vi "UHR-Fleezers Control (host) - 11.9b.vi"() -> ()   [LabVIEW 2014] (continued)
  out "Ave. Time (s)":dbl=7.5
  out "1 Channel":waveform(dbl)(graph)={"t0"=timestamp(0 s since 1904-01-01), "dt"=1.4999999999999999e-05, "Y"=array[20000 elements], "attributes"=variant("NI_ChannelName"=variant(string "T1 X"))}
  out "Slow mean":dbl=-0.0035457890155310146 format="%0.2f"
  in  "Slow mean N ave.":dbl=1.0 min=1.0 step=1.0
  out "Mean Intensity":dbl=-0.0035457890155310237
  out "Sigma":dbl=0.00558974165957254
  out "Sigma/Mean":dbl=-1.5764450831926926
  in  "Subtract mean":bool
  in  "High Res. Display":u16(ring)=1 items=["T1 Y", "T1 X", "T1 Sum", "T2 Y", "T2 X", "T2 Sum", "T1 FB X", "T1 FB Sum", "T2 FB X", "T2 FB Sum", "PSD Y", "PSD X", "PSD Y Sum"]
  out "APD 1 Rate (Hz)":dbl format="%#_3p"
  in  "Tab Control":T4(tab)
  in  "Red Laser ON/Interlacing":bool
  out "Good tether":bool
  out "Bad fit":bool
  in  "11":bool
  out "Stage Moving":bool
  in  "Read Cal":bool
  in  "Confocal\nLinescan":bool
  in  "Speed (nm/s)":dbl=100.0
  in  "Furthest Withdraw (MHz)":dbl=15.0
  in  "Confocal\nImage":bool
  in  "Round T1 X":bool caption="Round"
  in  "T1 offset_x (mV)":dbl=-22.37819181637641 format="%#_2g"
  in  "T1 k_x (pN/nm)":dbl=0.15700163781152213 min=0.0 step=0.001 format="%#_2g"
  out "Total Time (s)":dbl=60.0
  in  "Start Saving":bool
  in  "Cal sets to save":u32=25 min=1 step=1
  in  "Comment (data description)":string="testing confocal setup"
  out "Calibrating...":bool
  in  "Trap 2 (ON/OFF)":bool
  in  "Trap 1 (ON/OFF)":bool
  in  "Save Calibration":bool
  in  "N sets to save":u32=200 caption="N Sets"
  in  "Save N Sets":bool
  out "Save file name":path=path "E:/Data/120504/120504_125.dat"
  in  "Save ave N":dbl=250.0 caption="Averaging Factor"
  out "Saving...":bool
  in  "Stop Saving":bool
  out "Progress":u16(slide) scale=0.0..100.0
  out "Manipulating Trap":bool
  out "Buffer Status":dbl(slide) scale=0.0..1.0
  out "Overflow (data lost)":bool
  in  "Reset":bool
  out "Data Rate (Hz)":dbl=66666.66666666667 caption="Trap Data Rate (Hz)" format="%#_3p"
  out "Data Period (s)":dbl=1.4999999999999999e-05 caption="Trap Data Period (s)" format="%#_6p"
  out "Save Data Rate (Hz)":dbl=266.6666666666667 caption="Rate (Hz)" format="%#_6p"
  out "Save Data Period (s)":dbl=0.00375 caption="Period (s)" format="%#_6p"
  in  "T1 a_x (nm/V)":dbl=925.7792512885474 step=10.0 format="%#_3g"
  in  "T2 a_x (nm/V)":dbl=678.0121440160386 step=10.0 format="%#_3g"
  in  "T2 k_x (pN/nm)":dbl=0.2167951647771519 min=0.0 step=0.001 format="%#_2g"
  in  "T2 offset_x (mV)":dbl=-14.421148336697543 format="%#_2g"
  in  "BD 1 Frequency 1 (MHz)":dbl=67.75 caption="T1 X (MHz)" min=60.0 max=90.0 step=1.0 format="%#_6p"
  in  "BD 1 Frequency 2 (MHz)":dbl=83.0 caption="T2 X (MHz)" min=60.0 max=90.0 step=1.0 format="%#_6p"
  in  "Green ON/Interlacing":bool
  in  "Round T2 X":bool caption="Round"
  in  "AO1":dbl(slide)=5.0 caption="Confocal Y (V)" min=0.0 max=10.0 step=0.01 scale=0.0..10.0 scale format="%_1f"
  in  "AO2":dbl(slide)=5.0 caption="Confocal X (V)" min=0.0 max=10.0 step=0.01 scale=0.0..10.0 scale format="%_1f"
  in  "Trap Raster Scan":bool
  out "Raster Scanning...":bool
  in  "Trap D (MHz)":dbl=15.25
  in  "Setpoints (V)":cluster{"Set 1":dbl, "Set 2":dbl}={"Set 1"=9.0, "Set 2"=9.0}
  in  "Green FB Setpoint (mV)":dbl=90.0
  in  "Fish":bool
  out "Multiple tether":bool
  out "Hysteresis":bool
  in  "Target":bool
  in  "Active cal?":bool
  in  "Set Current\nPos to 0,0,0":bool
  in  "Position Label 5":string="Upper flow spot" caption="5"
  in  "Move to Position":bool
  in  "Position":dbl=1.0 min=1.0 max=10.0 step=1.0
  in  "Set Position":bool
  in  "Saved Stage Positions":dbl[][](array[numeric])=[[1.0, 0.0, 0.0, 0.0], [2.0, 0.47143, -1.65361, -0.02271], [3.0, 1.5, -0.5, 0.0], [4.0, -0.17227, -2.30048, -0.0394], [5.0, 1.5, -2.0, -0.02], [6.0, 0.0, 0.0, 0.0], [7.0, 0.0, 0.0, 0.0], [8.0, 0.0, 0.0, 0.0], [9.0, 0.0, 0.0, 0.0], [10.0, 0.0, 0.0, 0.0]]
  in  "Move to Position 5":bool
  in  "z nudge increment (um)":dbl=0.5
  in  "+z":bool
  in  "Position 1 Label":string="Lower capillary (DNA beads)" caption="1"
  in  "Set Position 1":bool
  in  "Set Position 2":bool
  in  "Set Position 3":bool
  in  "Set Position 4":bool
  in  "Move to Position 3":bool
  in  "Move to Position 4":bool
  in  "Move to Position 2":bool
  in  "Move to Position 1":bool
  in  "Position 2 Label":string="Upper capillary (ADig beads)" caption="2"
  in  "Position 3 Label":string="Lower flow spot" caption="3"
  in  "Position 4 Label":string="Dump beads" caption="4"
  in  "-z":bool
  in  "Set Position 5":bool
  out "Stage Control Serial Error":errorcluster
  in  "Use Harvard pumps\nfor beads (else Chemyx)":bool=TRUE
  in  "Tab Control 9":enum32{"Harvard Pumps", "Chemyx Pumps"}(tab)
  in  "Normal volume (mL)":dbl=200.0
  out "Samp flush bar":dbl(slide)=0.8066666666666666 scale=0.0..1.0
  out "Flushing samp":bool caption="Flushing"
  out "P1 Flush Volume (uL)":dbl=100.5 caption="Volume (mL)"
  out "P3 Flush Volume (uL)":dbl=121.0 caption="Volume (mL)"
  out "P3 Flushing Bar":dbl(slide)=0.8066666666666666 scale=0.0..1.0
  in  "Display On P3":bool caption="Display On"
  in  "Normal Flow Rate (ul/h) P3":dbl=800.0 caption="Normal Flow Rate (ml/h)"
  out "Flushing P3":bool caption="Flushing"
  in  "Retract Vol 1 (uL)":dbl=50.0 caption="Volume (mL)"
  in  "Retract Vol 3 (uL)":dbl=100.0 caption="Volume (mL)"
  in  "Retract Rate (mL/m)":dbl=2000.0
  in  "Retract Pump 1":bool
  in  "Retract Pump 3":bool
  in  "Stop Flow":bool
  in  "Start Flow":bool
  in  "Flush Sample":bool
  in  "Flush volume (mL)":dbl=100.0
  in  "Flush rate (mL/m)":dbl=100.0
  in  "Normal Flow rate (mL/h)":dbl=100.0
  in  "Clear Volume":bool caption="Clear Infused Volume"
  in  "Flush Pump 3":bool
  in  "Volume (uL) P3":dbl=150.0 caption="Volume (mL)"
  in  "Flush rate (uL/m) P3":dbl=100.0 caption="Rate (mL/m)"
  out "Flushing P1":bool caption="Flushing"
  in  "Volume (uL) P1":dbl=100.0 caption="Volume (mL)"
  in  "Flush rate (uL/m) P1":dbl=100.0 caption="Rate (mL/m)"
  in  "Normal Flow Rate (ul/h) P1":dbl=600.0 caption="Normal Flow Rate (ml/h)"
  in  "Flush Pump 1":bool
  in  "Clear Volume P3":bool caption="Clear Infused Volume"
  in  "Clear Volume P1":bool caption="Clear Infused Volume"
  in  "Display On P1":bool caption="Display On"
  out "P1 Flushing Bar":dbl(slide)=1.005 scale=0.0..1.0
  out "Samp Volume (uL)":dbl caption="Volume (mL)"
  out "Total Volume\nFlowed P1 (uL)":dbl caption="Total Volume\nFlowed (mL)"
  out "Total Volume\nFlowed P3 (uL)":dbl caption="Total Volume\nFlowed (mL)"
  out "Total Volume\nFlowed Samp (uL)":dbl caption="Total Volume\nFlowed (mL)"
  in  "All Pump Parameters":T5={"Pump 1"={"Diameter (mm)"=4.61, "Units"=4.0, "Volume"=100.0, "Rate"=25.0}, "Pump 2"={"Diameter (mm)"=4.61, "Units"=3.0, "Volume"=0.0, "Rate"=0.0}, "Pump 3"={"Diameter (mm)"=4.61, "Units"=4.0, "Volume"=100.0, "Rate"=800.0}}
  in  "Total Volume\nFlushed (uL)":dbl
  in  "Inject Pump 2":bool caption="Inject Pump 2\n(Flush Center)"
  in  "Flush Center Ch Rate (ul/m)":dbl=100.0
  in  "Flush Center Ch Volume (uL)":dbl=15.0
  in  "Pump pause delay (ms)":u32
  in  "Pump write delay (ms)":dbl=300.0
  in  "Ch 3 Inject Rate (ul/h)":dbl=800.0
  in  "Ch 3 Inject Volume (uL)":dbl=100.0
  in  "Ch 1 Inject Volume (uL)":dbl=100.0
  in  "Ch 1 Inject Rate (ul/h)":dbl=25.0
  out "Pump 1 cont disp":string="Right: DNA beads "
  out "Pump 3 cont disp":string="Left: ADig beads"
  in  "Read Harvard":bool
  out "read buffer":string
  out "Serial Settings:Number of Bytes at Serial Port":u32
  in  "write buffer":string
  in  "Tab Control 2":T6(tab)=enum."Feedback on Trap Position"
  out "Total Counts (ticks)":u32=600
  in  "Trap ON/OFF X or Y Amp?":bool=TRUE
  in  "Oscillate Set 1":bool
  in  "Trap 1 ON":bool
  in  "Number Interlace Sets":u8=3 min=1 max=3
  in  "DIO count 3 (ticks)":u32=200
  in  "DIO count 2 (ticks)":u32=200
  in  "DIO count 1 (ticks)":u32=200
  in  "BD 2 Amplitude 3 (%)":dbl min=0.0 max=50.0 step=1.0
  in  "BD 2 Amplitude 2 (%)":dbl min=0.0 max=50.0 step=1.0
  in  "BD 2 Amplitude 1 (%)":dbl min=0.0 max=50.0 step=1.0
  in  "BD 1 Amplitude 3 (%)":dbl min=0.0 max=50.0 step=1.0
  in  "BD 1 Amplitude 2 (%)":dbl=35.0 min=0.0 max=50.0 step=1.0
  in  "BD 1 Amplitude 1 (%)":dbl=10.0 min=0.0 max=50.0 step=1.0
  in  "BD 2 Frequency 3 (MHz)":dbl=26.0 min=0.0 max=40.0 step=1.0 format="%#_6p"
  in  "BD 1 Frequency 3 (MHz)":dbl=70.0 min=60.0 max=90.0 step=1.0 format="%#_6p"
  in  "BD 2 Frequency 2 (MHz)":dbl=26.0 min=0.0 max=40.0 step=1.0 format="%#_6p"
  in  "BD 2 Frequency 1 (MHz)":dbl=26.0 min=0.0 max=40.0 step=1.0 format="%#_6p"
  in  "Not-Interlacing Set":enum32{"Set 1", "Set 2", "Set 3"}(radio)
  in  "Interlace":bool=TRUE
  in  "Trap 2 ON":bool
  in  "Trap 3 ON":bool
  in  "Scan axis 2":bool=TRUE
  in  "Osc. freq. (Hz)":dbl=0.25
  in  "Osc. amp. (MHz)":dbl=2.0
  out "Coords":T7
  in  "Manipulation Scaling":cluster{"Horizontal":dbl, "Vertical":dbl}={"Horizontal"=0.075, "Vertical"=0.01}
  in  "Freq or Amp switch first":bool=TRUE
  in  "Swap F1 and F2":bool
  in  "Freq switch delay":u16
  in  "Amp switch delay":u16=5
  in  "MCL Step Increment (V_int)":dbl=3.0
  out "Time to Finish All (min)":dbl=0.15651 format="%#_2p"
  in  "Scan Speed (nm/s)":dbl=100.0
  in  "Scan Range (nm)":dbl=470.0
  in  "Step Size (nm)":dbl=1.0
  in  "MCL/AOM Scale Tweak":dbl=1.0
  in  "MCL Step Position Ratio":dbl=0.5
  in  "Move MCL Also?":bool=TRUE
  out "Final sep (nm)":dbl=1520.75
  out "Initial sep (nm)":dbl=1050.75
  out "Save index":dbl=125.0
  out "Final D (MHz)":dbl=19.071138211382113
  out "Initial D (MHz)":dbl=15.25
  out "Final freq. (MHz)":dbl=63.92886178861789
  out "Initial freq. (MHz)":dbl=67.75
  in  "Saved AOD Raster Scan Parameter Sets":T8(array[cluster])=[{"Scan Range AOD (nm) 2"=500.0, "Step Size AOD (nm) 2"=1.0, "Scan Speed AOD (nm/s) 2"=100.0, "Number of scans (AOD) 2"=1, "Label"="offset curve"}, {"Scan Range AOD (nm) 2"=450.0, "Step Size AOD (nm) 2"=1.0, "Scan Speed AOD (nm/s) 2"=100.0, "Number of scans (AOD) 2"=1, "Label"="hp raster check"}, {"Scan Range AOD (nm) 2"=6.8, "Step Size AOD (nm) 2"=0.34, "Scan Speed AOD (nm/s) 2"=0.34, "Number of scans (AOD) 2"=1, "Label"="3.4 kbp - 1 bp steps"}, {"Scan Range AOD (nm) 2"=215.0, "Step Size AOD (nm) 2"=1.0, "Scan Speed AOD (nm/s) 2"=100.0, "Number of scans (AOD) 2"=3, "Label"="dt14 1 14 MHz start"}, {"Scan Range AOD (nm) 2"=450.0, "Step Size AOD (nm) 2"=1.0, "Scan Speed AOD (nm/s) 2"=100.0, "Number of scans (AOD) 2"=1, "Label"="dt14 2 small beads"}, {"Scan Range AOD (nm) 2"=470.0, "Step Size AOD (nm) 2"=1.0, "Scan Speed AOD (nm/s) 2"=100.0, "Number of scans (AOD) 2"=1, "Label"="Oligo"}, {"Scan Range AOD (nm) 2"=410.0, "Step Size AOD (nm) 2"=1.0, "Scan Speed AOD (nm/s) 2"=100.0, "Number of scans (AOD) 2"=1, "Label"="hp raster check"}, {"Scan Range AOD (nm) 2"=650.0, "Step Size AOD (nm) 2"=1.0, "Scan Speed AOD (nm/s) 2"=100.0, "Number of scans (AOD) 2"=1, "Label"="Monika"}, {"Scan Range AOD (nm) 2"=1000.0, "Step Size AOD (nm) 2"=1.0, "Scan Speed AOD (nm/s) 2"=100.0, "Number of scans (AOD) 2"=1, "Label"="Monika offset"}]
  in  "Load parameters":bool
  out "Scan Range (MHz)":dbl=-3.821138211382114
  in  "Restart DMA? (AOD)":bool=TRUE caption="Restart DMA?"
  out "Incr. int (AOD)":i64=-7759651845
  out "Time/Scan (s) (AOD)":dbl=4.6953000000000005 format="%#_2p"
  out "Data points/scans":dbl=626040.0
  out "Data points/scan (f/b)":dbl=626040.0
  in  "Save scans":bool=TRUE
  out "AOD Scan I":u64 caption="Scan I"
  in  "Continuous AOD Scanning":bool caption="Continuous Scanning"
  in  "Abort AOD Scan":bool caption="Abort Scan"
  in  "Scan BD":bool=TRUE
  out "Cycles/step (AOD)":u64=666 format="%.3p"
  in  "Number of F/B Scans (AOD)":u16=1 min=1
  out "Scan steps (AOD)":u64=470
  out "Scan Increment (MHz)":dbl=-0.00814741622895973
  out "AOD Scanning":bool caption="Scanning"
  in  "Start AOD Scan":bool caption="Start Scan"
  out "N sets should be saved":dbl=31.302
  out "Progress 2":u16(slide) caption="Progress" scale=0.0..100.0
  in  "Abort save 2":bool caption="Abort save"
  in  "Trap 1 Bead Size (nm)":dbl=860.0
  in  "Trap 2 Bead Size (nm)":dbl=790.0
  out "MCL Count":dbl=782931.6080202644
  in  "All FB On/Off":bool=TRUE
  in  "AI2 to Setpoint":cluster{"Set 1":bool, "Set 2":bool}
  out "AI2 (V)":cluster{"Set 1":dbl, "Set 2":dbl}={"Set 1"=-0.0027466658528397473, "Set 2"=-0.0030518509475997192}
  in  "Reset Feedback":cluster{"Set 1":bool, "Set 2":bool}
  in  "PID Gains":T9={"Set 1"={"proportional gain (Kc)"=0, "integral gain (Kc*Ts/Ti)"=5, "derivative gain (Kc*Td/Ts)"=0}, "Set 2"={"proportional gain (Kc)"=0, "integral gain (Kc*Ts/Ti)"=5, "derivative gain (Kc*Td/Ts)"=0}}
  in  "Feedback On/Off":cluster{"Set 1":bool, "Set 2":bool}={"Set 1"=TRUE, "Set 2"=TRUE}
  in  "Rem fb disp offset":bool caption="Rem. Offset"
  in  "Remove Offset to factor":bool
  in  "FB Trap Pos Offset":dbl=-9.744913000168507 caption="Offset (nm)" format="%.1f"
  in  "Negate Y Axis":bool=TRUE
  in  "Set Reading to\nSetpoint":bool
  out "Trap X (AI1)":T10={"Trap 1"=0.29998779296875, "Trap 2"=0.399993896484375}
  in  "Trap Pos FB SP":fxp<+/-,16,1>=-0.10723876953125 caption="Setpoint"
  in  "Trap Pos. FB ON":bool
  in  "Reset Trap Pos. FB":bool
  out "Trap Positions":waveform(dbl)[](graph)=[{"t0"=timestamp(13.800000000000011 s since 1904-01-01), "dt"=0.15, "Y"=[-9.744913000165011, -9.744913000165011], "attributes"=variant("NI_ChannelName"=variant(string "Trap 1 Pos."))}, {"t0"=timestamp(13.800000000000011 s since 1904-01-01), "dt"=0.15, "Y"=[-3.495870259939693e-12, -3.495870259939693e-12], "attributes"=variant("NI_ChannelName"=variant(string "Trap 2 Pos."))}]
  in  "Tab Control 8":enum32{"Main Setting", "Details"}(tab)=enum."Details"
  in  "Green Laser ON/OFF":bool
  in  "Offset SP2 from SP1":bool
  in  "Use SP 2":bool
  in  "Trap Pos FB Int Count":u16=100
  in  "Trap Pos. FB Gains":T11={"proportional gain (Kc)"=10.0, "integral gain (Kc*Ts/Ti)"=10.0, "derivative gain (Kc*Td/Ts)"=0.0} {"proportional gain (Kc)" format="%.11g"; "integral gain (Kc*Ts/Ti)" format="%.11g"; "derivative gain (Kc*Td/Ts)" format="%.11g"}
  in  "Trap Pos FB SP 2":fxp<+/-,16,1>=-0.10723876953125 caption="Setpoint 2"
  in  "SP2 Offset":fxp<+/-,16,1>=0.100006103515625
  in  "Negate Diff?":bool=TRUE
  in  "Differential FB?":bool=TRUE
  in  "Trap Pos. FB Offset Factor":i64
  in  "Trap Pos FB Negate Action":bool
  in  "Trap Pos. FB Mult Factor":i64=16777216
  in  "Trap Pos. AI1 X Pre-scale":u16
  in  "Trap Pos. FB Range":T12={"output high"=0.999969482421875, "output low"=-1.0}
  out "Trap Pos FB Int Signal":fxp<+/-,24,9>=-2.007537841796875 format="%.18g"
  out "Trap Pos FB Int-Norm Signal":fxp<+/-,16,1>=-0.02008056640625 format="%.16g"
  in  "Set SP Using...":bool
  in  "Trap Pos FB Monitor\nT1 or T2":bool
  out "Trap X AI1 (DMA)":T13={"Set 1"=-1.0, "Set 2"=-1.0}
  in  "N El. to Ave.":dbl=10000.0
  out "Trap Pos FB Action":i64
  out "Action (%)":dbl(knob) scale=-100.0..100.0
  in  "Trap Pos. FB Out Scale 2^n":u8=24 caption="Action Scale Factor"
  out "Mean T1 Position (nm)":dbl=-9.744913000165011 caption="Mean T1 (nm)" format="%0.2f"
  out "Trap 1 Position RMS (A)":dbl caption="RMS (Å)"
  in  "Remove Action Offset":bool
  in  "factor":dbl=0.8
  in  "Trap Pos. Disp. Downsample":dbl=10000.0 caption="Trap Downsample"
  in  "Tab Control 3":enum32{"Timing", "MCL Scan", "Analog Out"}(tab)
  out "APD 2 Gate Late Counter":u32
  out "APD 2 Gate Relative Phase":i16
  in  "Phase Adj. (APD 2 Gate)":i16=20
  in  "Initial Phase Adjustment (APD 2 Gate)":i16=55
  out "APD 1 Gate Late Counter":u32
  in  "- phase (APD 1 Gate)":bool
  in  "+ phase (APD 1 Gate)":bool
  out "APD 1 Gate Relative Phase":i16
  in  "Phase Adj. (APD 1 Gate)":i16=20
  in  "Initial Phase Adjustment (APD 1 Gate)":i16=60
  in  "Save APD Data\nwith Trap Data":bool=TRUE
  out "APD FIFO Elements Remaining":u32
  in  "- phase (APD Acq)":bool
  in  "+ phase (APD Acq)":bool
  out "APD Acq Late Counter":u32
  out "APD Acq Relative Phase":i16
  in  "Phase Adj. (APD Acq)":i16=20
  in  "Initial Phase Adjustment (APD Acq)":i16
  in  "Invert APD Gate":bool caption="Invert Gate"
  in  "APD Gate OFF Count":u32=450 caption="Gate OFF Count"
  in  "APD Gate ON Count":u32=150 caption="Gate ON Count"
  in  "APD Gate":enum32{"ON", "OFF", "Interlace"}(radio)=enum."Interlace"
  in  "APD Integration Time (s)":dbl=0.01 caption="Integration Time (s)"
  out "APD Acq Rate (Hz)":dbl=100.0 caption="Rate (Hz)"
  out "APD Samples/FIFO Acq.":dbl=30.0
  out "APD Elements/DMA read":u32=60
  out "APD Int. Count":u32=400000 format="%.0p"
  in  "+ phase (APD 2 Gate)":bool
  in  "- phase (APD 2 Gate)":bool
  in  "Tab Control 5":enum32{"PSD X", "PSD Y", "Other Data Channel"}(tab)
  out "Data map":dbl[][](graph)=[[-0.009093117685790525, -0.007930362371143508, -0.007754257275205968, -0.008007549817249278, -0.007602052846338941, -0.007912268435502932, -0.007607960084622785, -0.0075511280459739025, -0.0075659235273027765, -0.008250603527173198, -0.00813251622962637, -0.008594668588708203, -0.009399585249933565, -0.007647222257289099, -0.009101202856383231, -0.008282046280890548, -0.009811094602988905, -0.00756717949318091, -0.009140567007915868, -0.0073843309806302946], [-0.008493807361303536, -0.007663617072649492, -0.008256205022532336, -0.007952830185196302, -0.007279874418184582, -0.007356798116565186, -0.0069743489143222585, -0.007520087991651134, -0.007361850724229795, -0.007389116586560407, -0.007775790827289851, -0.008683184943784783, -0.008790211727097149, -0.007806810616736395, -0.008982907777700291, -0.007650155522875499, -0.009388247877714903, -0.007552137445539828, -0.008977826950618533, -0.007886203299123228], [-0.008181893320929307, -0.00839471338042945, -0.007799952401828855, -0.008308044384906312, -0.008275645030715005, -0.007401990323496574, -0.006875323319245371, -0.0070218178801166025, -0.006512198698798073, -0.0063178688570392095, -0.006805180239267433, -0.007518346532565596, -0.008735692049743055, -0.00724608634970231, -0.008704712767052859, -0.007945321438686287, -0.008767860926849669, -0.007671020451478872, -0.00875386344445876, -0.007695295089867138], [-0.008130119935988365, -0.007136557696350718, -0.007373598169435823, -0.007233072138047845, -0.0077281747998472865, -0.005849249829228351, -0.005735947777185798, -0.004739559736975043, -0.004920183410197928, -0.0038166885698606785, -0.004682785911972345, -0.005039020484130334, -0.00690087468071523, -0.006215680179303547, -0.0074666456406588646, -0.00814641889723231, -0.008228414513586805, -0.0073042911866212775, -0.008535443147109325, -0.007689317045800068], [-0.008048339688765222, -0.0070262103984282814, -0.006784428381835994, -0.006462947020101757, -0.005413544226518168, -0.0028972309457726553, -0.002613656344091552, -0.0007913579983610413, -0.0010255539568848066, 0.0006448033640966027, -0.0005086805713629527, -0.001297083649014534, -0.003337801791559313, -0.002740630934904912, -0.005540289041049259, -0.006466196037469115, -0.007893084684782161, -0.007253383480927094, -0.008523649067154491, -0.008424970867227096], [-0.008692622082261615, -0.007319521217364842, -0.005755111221817798, -0.003792540532687189, -0.00227942708102312, 0.000483266681506554, 0.0014973802606671, 0.003540650121447641, 0.004028332480785218, 0.005135244197648001, 0.003981153966581634, 0.0034636396067710545, 0.0017501855516850323, 0.0010275870097429896, -0.0024058090542775825, -0.004619508847101628, -0.00696689371632374, -0.006931245628688383, -0.008182025780859851, -0.007815950695329976], [-0.00821540874240863, -0.005867179558433026, -0.0038147206017466926, -0.0012540547752299272, 0.0009272510857660976, 0.004482725069077296, 0.005094761342461562, 0.006396333111961989, 0.006641489865394995, 0.008244873838360105, 0.00622024214014944, 0.005437421631898459, 0.0037062196383043787, 0.0039079284440514134, 0.00011910739683561111, -0.0021155745359372523, -0.0052920825878262235, -0.006269707480838847, -0.00771057032521053, -0.007948241106374241], [-0.007884864746179087, -0.005659354512526344, -0.002544916655066751, 9.730381565131179e-05, 0.0019679392499950933, 0.003980498813834972, 0.004545595176909105, 0.005211998880279077, 0.004316308793345271, 0.0049582106101100296, 0.004417272839063756, 0.004152457319364951, 0.0028044785889019025, 0.00406546833676348, 0.0004537962268733079, -0.0022503305680760134, -0.004833591485740649, -0.005815590438963289, -0.006409661910137404, -0.00747004429812991], [-0.007583267382238386, -0.004882000882934762, -0.0038451140355032776, -0.0016369446668547012, -0.0012364145574272002, 0.00024560570156679373, 0.0001795553469662146, 0.00059301095989026, -0.0004598253721832719, 0.0006432265077103554, -0.0005366492251270509, -0.00024492525087133033, -0.0008478979763931471, 0.0004355022865183716, -0.002224596882477229, -0.0030354619889501723, -0.005565311948490649, -0.006021505826488022, -0.0069210753467628845, -0.007879944918476524], [-0.008040346878090326, -0.006862696971498104, -0.006336491878674995, -0.005461350586097968, -0.005940054654849293, -0.004512649878881008, -0.005018950037994686, -0.0043380418634407164, -0.004709873373528969, -0.004442153494476381, -0.005131912732517138, -0.004937093503234647, -0.006064322362111088, -0.004728773424951794, -0.006301422293530947, -0.006624384767080079, -0.008081381277763696, -0.00789390592402444, -0.007979806702532219, -0.007895618667850521], [-0.009072596458312808, -0.00880289426096623, -0.0092848563929495, -0.010326479907538676, -0.010798822549107683, -0.009119956258571284, -0.009276114327973069, -0.009089354383039431, -0.009417098163877372, -0.009282915028834361, -0.010344781966702844, -0.009775595105550903, -0.010376003571655317, -0.01021568866775812, -0.011229840225717491, -0.010464341733335863, -0.010657278856759583, -0.009430048577759108, -0.009007295643070796, -0.008342923163363568], [-0.010032577110923473, -0.01048419830062017, -0.01247741022526665, -0.013958311167976727, -0.014919942316729927, -0.014408175422791913, -0.014103923396234723, -0.014744110243936143, -0.014993684986384455, -0.014308447607056084, -0.014937884607659595, -0.015720355253606696, -0.01581234985152132, -0.015517778210244481, -0.01570381347938231, -0.014005181025264823, -0.012564060007705888, -0.01019230034187177, -0.00996108339473993, -0.009007894716188836], [-0.01015831765102569, -0.011625066910300597, -0.013873555893446923, -0.01642046988438768, -0.01850466093024781, -0.019125349960614338, -0.018875498399497426, -0.018924030983383168, -0.02003782808665338, -0.019680135464925662, -0.0199962216477468, -0.02075322752078982, -0.021393804340805025, -0.01892377236854445, -0.017709124629425012, -0.015373965133689256, -0.012883748138151182, -0.011135266972937988, -0.01001563256802752, -0.009346177295655143], [-0.010235131581835623, -0.010548350660948624, -0.01319737955485069, -0.0170756093956873, -0.019682853747901498, -0.021422463301004592, -0.023065732990637723, -0.02311157923810582, -0.02400703774239577, -0.024058458246623678, -0.0240676102995906, -0.02454338695921686, -0.023059059168390954, -0.02006456011149576, -0.017542880027533084, -0.015594551823595627, -0.012758502028002598, -0.010692028843963627, -0.009120734769953582, -0.009382803853976038], [-0.00927124611976432, -0.010163129942715295, -0.012001835840693881, -0.015492617365098072, -0.01804371733697946, -0.020276281639691262, -0.02249444284045994, -0.02399581278990765, -0.02410995799246074, -0.024520143091590986, -0.024440837449861495, -0.023755329314732447, -0.02173444185100297, -0.01888988196650751, -0.015717316137677406, -0.01330102590922941, -0.010307393064907727, -0.009992927689312977, -0.008948368344090785, -0.009171185426330289], [-0.008913670110033758, -0.009487748541153324, -0.010271220953760277, -0.012822685168547666, -0.014877933408246618, -0.01645708382270735, -0.018174418710522888, -0.02006592401438696, -0.020560245735494094, -0.020880445185878234, -0.019757749059474437, -0.019731420523350106, -0.01748349679551805, -0.014933401179938435, -0.01287075469100105, -0.012375615253101852, -0.01017571614409014, -0.010194053140322132, -0.008327555288192647, -0.009296945225881956], [-0.008651703429240758, -0.00859123261526902, -0.0087124516001243, -0.010702988201589679, -0.011158446775450175, -0.013551662787714375, -0.013899713264433188, -0.015139676175909094, -0.015358154174100445, -0.01585371404194936, -0.015240285383275445, -0.015633640866232926, -0.013444202320888608, -0.012235117407072522, -0.010180277760900221, -0.010599065418614181, -0.008836891782999633, -0.009612080137946436, -0.008061008352690049, -0.008692954060992533], [-0.008978999428748309, -0.00853630494854542, -0.008448003588981772, -0.009555269362758849, -0.009800170309108366, -0.010532180047368476, -0.011577191415346372, -0.012522786451981825, -0.011897509550792433, -0.012765293465086206, -0.012382882546317676, -0.012580658559524002, -0.011517787256641054, -0.011479669503957436, -0.009468386619803586, -0.009506617110587617, -0.008814998176882461, -0.008907308155253858, -0.008359272542371161, -0.007728018696215012], [-0.008567772547654876, -0.009179160254178084, -0.008797883700935975, -0.008966540233807333, -0.009244399721063817, -0.010241100172431, -0.009683978551547411, -0.010741416747860222, -0.010801534838144658, -0.011948471067133912, -0.010638943408897612, -0.011276692781352033, -0.010482972789145662, -0.009951530542563796, -0.008872861351211857, -0.009011466300733673, -0.008130228774171959, -0.008497529899096853, -0.008537094090014226, -0.008554927038672385], [-0.00883740874692164, -0.008522568147033945, -0.008057007463930647, -0.00857500256200953, -0.00892333639038801, -0.0102483493423614, -0.009382806505145502, -0.010288681907090315, -0.009776552705287204, -0.010709303069246771, -0.009812157424141538, -0.011540991338011664, -0.009448072118884751, -0.009215522072108621, -0.007990643964211522, -0.00861551413050941, -0.008069591988205893, -0.008448705150511306, -0.008173872666663988, -0.0077366764957025325], [-0.00866188543514634, -0.00837290321697088, -0.007616576548930206, -0.008620554974306619, -0.008879342477325386, -0.009976131360122594, -0.009197328720787731, -0.010891970058339532, -0.009831409253817102, -0.010963285150790543, -0.00943682713188495, -0.010250758011437967, -0.009316627581118588, -0.008698498423952166, -0.007894210972856612, -0.008627558747470431, -0.008684295707717409, -0.008540742057574494, -0.008058236803640907, -0.008796687176971204], [-0.008960243147743728, -0.008389810955552138, -0.00847348274282588, -0.008961453295347137, -0.008457770304110886, -0.00929036551389055, -0.008754051280419149, -0.010523443067409842, -0.009918731765266534, -0.010037112915448395, -0.0094884291794276, -0.009837286274472896, -0.008576890056086488, -0.008579749000379288, -0.0076704608190795035, -0.008975965021771925, -0.00787633064191945, -0.008529814016465537, -0.008210449633173293, -0.00923149421792313], [-0.008958509491948936, -0.0079752458499608, -0.007575580767324844, -0.008803256661217552, -0.008651176181790142, -0.009290225911366488, -0.008694199017275235, -0.00928758206050638, -0.008685080197252814, -0.009895043342157074, -0.008890181034455161, -0.009708286739414866, -0.008159548355032305, -0.008011065029368486, -0.007472994792829198, -0.008178707159361769, -0.008186872200841244, -0.008748187311294335, -0.008332749653614566, -0.009032986118264676], [-0.008984454676541142, -0.008385860780740762, -0.008233303603375429, -0.008883308711661035, -0.008263391222137696, -0.008615507326621034, -0.008345881820440536, -0.009360059323812333, -0.008525712363877502, -0.00936688813432775, -0.008501006453744242, -0.009857020401666132, -0.008518026774209042, -0.008466286706819728, -0.007595230844466895, -0.008637429843490887, -0.008247148821298463, -0.009757163330206205, -0.008351945487579443, -0.008826303902292224], [-0.008793473634059202, -0.008532826676629766, -0.008301057942882255, -0.007918519844410386, -0.008166427002916622, -0.008334776051627416, -0.008198383116294311, -0.008466661691906446, -0.008900494330306541, -0.009018032342304892, -0.008921561030554092, -0.00970008519907525, -0.00858060303466588, -0.008488668571179206, -0.008067629578802802, -0.009301914211857531, -0.007584888207047696, -0.009401246667708162, -0.00838952961198379, -0.009295622811186042], [-0.008612970994324173, -0.009228313227038376, -0.008109777026918365, -0.007900894002180022, -0.008577211653308246, -0.0078092842189432105, -0.009066038409420633, -0.008632114747530527, -0.00915628345868762, -0.009033529956806095, -0.008473548831738616, -0.009753001297439137, -0.008794013472457105, -0.009389760586935149, -0.008294543199585239, -0.009165299461629816, -0.0080445379542478, -0.01003357859191055, -0.008128570719288741, -0.009697938695473063], [-0.00842310878053087, -0.009238538415546935, -0.00789546954167132, -0.007785705695342489, -0.009075128619983087, -0.008134761036174236, -0.009034531715798766, -0.009110522965510081, -0.009372563691683431, -0.00973005869285193, -0.00918442879120475, -0.010224588766867198, -0.009149068560019315, -0.009118548250909013, -0.008665028583165667, -0.009663782970913627, -0.00822885864974483, -0.009561747582651057, -0.007796335718971677, -0.009448741371668462], [-0.008678814702107202, -0.008811871163062448, -0.008591634991878266, -0.008380498253149257, -0.008708521567010137, -0.009080766138792232, -0.009201278029004847, -0.009050300838444577, -0.00961322000266123, -0.009519398380897704, -0.009289741534829938, -0.010063257530557933, -0.009451879246656355, -0.009483739594157017, -0.008678484677225835, -0.00990455006759744, -0.00828239408358521, -0.009970239333168224, -0.008374145539585563, -0.009350844619784601], [-0.008045661641927443, -0.008394412754688788, -0.008552414855659416, -0.009271231425342906, -0.009328147806528048, -0.009046283727420858, -0.009056500460447304, -0.009214165466210778, -0.008945766230968395, -0.009389003022486266, -0.009144492868201123, -0.010147409487001281, -0.009339702713667958, -0.009380077870026074, -0.00835831230057397, -0.009990575898077645, -0.00854232985662241, -0.010366719217208723, -0.008640298575886954, -0.009403613854008858], [-0.008906889127393642, -0.00883118612173188, -0.008453805334277639, -0.00911933095261894, -0.00944887473163078, -0.010310422619086147, -0.009422604595844552, -0.009605385777620547, -0.008426093890224026, -0.01002127148121337, -0.009163459766844236, -0.009814776920437831, -0.008805402929197629, -0.009061616458602838, -0.008487717951513573, -0.009191908002197161, -0.00895972804734331, -0.009660499045960346, -0.008531815925380855, -0.009156879524597247], [-0.008741790054105969, -0.008549257028348849, -0.008797177164368942, -0.009662615006030037, -0.009307487432021831, -0.010322476933490709, -0.008290986210407227, -0.009590805326173235, -0.008934433308237403, -0.009471594992405057, -0.009687824691862398, -0.008931649605826689, -0.008484875544949318, -0.008583409860835651, -0.008351995170223395, -0.009053355535672075, -0.008484405156741804, -0.009874981465109369, -0.008438016030919395, -0.008858275353968496], [-0.00856709491696853, -0.00871265258961926, -0.007921953758409758, -0.009438005293459928, -0.008790640173333714, -0.0093055027234527, -0.008862492730787506, -0.009554208136696149, -0.008482487683988672, -0.01056028798055526, -0.009019149534255914, -0.010050471464200648, -0.00853462219965744, -0.009035449977530046, -0.008112572868495047, -0.008163535201347372, -0.008202407620730396, -0.008747092382002523, -0.00884982609053558, -0.008679668249538044], [-0.008394092371377686, -0.008489154891055648, -0.007659112578658681, -0.00902617957109932, -0.008357595543619473, -0.00961141464742498, -0.008884930906477895, -0.009113321109040815, -0.008880712493923793, -0.010292101237114604, -0.008975496191390358, -0.009710498384115248, -0.008935238162886418, -0.008502221359307316, -0.007752007669347329, -0.007720289124192612, -0.00788689558570684, -0.009181183359262636, -0.00856116046669701, -0.008611585911764589], [-0.008107502655444382, -0.008803676635770773, -0.008830636807290671, -0.008630461742231518, -0.008271369463273916, -0.009203900561491018, -0.008405901304371377, -0.009465853346718931, -0.008950045768193703, -0.009917010857616374, -0.008801581772901624, -0.010150568437297405, -0.008851987437577317, -0.00849255435289463, -0.007881778453429272, -0.007697298607360614, -0.007699527977878644, -0.008589254525886943, -0.007882418667869784, -0.007557576864658732], [-0.008427126089052106, -0.008873246741217405, -0.007984509944572782, -0.008215086829640958, -0.008087204687383241, -0.008627825617963911, -0.008679915351090582, -0.008599184356607833, -0.008277243783790082, -0.009885402202754485, -0.008578730059413158, -0.009265716716539838, -0.008533719952427615, -0.008773683534694161, -0.00758856120767947, -0.008144086881928147, -0.008079560975909644, -0.008313965537627473, -0.008565002742326862, -0.008110889204162412], [-0.008120547360555588, -0.008248284005375792, -0.007905963350631368, -0.008299804257910725, -0.007514734008193604, -0.008466861391934699, -0.007969212201198558, -0.007888984029732645, -0.008696999162581685, -0.009067749176828406, -0.008736340056677103, -0.008654004998204434, -0.008344040713692526, -0.008594741510905897, -0.0074614182850967405, -0.008103078495185257, -0.008057187148527191, -0.008974257694279996, -0.008197872328626302, -0.0074028505391394404], [-0.008307364139471399, -0.00821873274915887, -0.007970649657121935, -0.00815826403385205, -0.008457049180131213, -0.008316579982009714, -0.00790309541305004, -0.007939607987239819, -0.008478315283633124, -0.008288272322383177, -0.009147562816129263, -0.008684972824515615, -0.008675749750533264, -0.007960612097219584, -0.008024961861627669, -0.008590987458143061, -0.007831114204848427, -0.009273090840284501, -0.007678985566660499, -0.008250217200435749], [-0.008439006720363235, -0.008607324538260196, -0.008928480199152027, -0.00907069045095883, -0.008371906943686698, -0.00843318137977436, -0.007928947055533257, -0.008211444982725611, -0.007814800246802284, -0.008561224417862523, -0.0083263104139755, -0.00864694388438663, -0.008317511287294722, -0.008392142509562009, -0.0080180144415389, -0.00841215643506122, -0.008129752772469346, -0.009147606927106531, -0.008461182057229562, -0.008704070030515779], [-0.008805306104753604, -0.008527006486683296, -0.008608832647163441, -0.008197721113858471, -0.008101085524828317, -0.008548783050390606, -0.008327728211326255, -0.00811669551471623, -0.007841959263305661, -0.008369922080743528, -0.007863509709325214, -0.008398594443287834, -0.008357926530931568, -0.007776338967419011, -0.00761957377022411, -0.00797846909846784, -0.00760217145174542, -0.009062943091421194, -0.008736809526389501, -0.009068120509011127], [-0.008594961447082165, -0.00896668650229153, -0.008417303751339367, -0.008410738059004663, -0.008191514788819833, -0.008993325778492794, -0.008023878772254618, -0.008285263880744707, -0.00783265428172105, -0.0073528870683615775, -0.008791245239786302, -0.00865234690848487, -0.008338402850135743, -0.00784027413088714, -0.007823138263178549, -0.007490285631650851, -0.008212733160155018, -0.008264156227590665, -0.008446206631865719, -0.00904272930587351]]
  in  "Channel":i32=4
  in  "Abort MCL Scan":bool
  out "MCL Scan I":u64
  out "MCL Scanning":bool
  in  "Start MCL Scan":bool
  out "wait to reset values":bool
  in  "Tab Control 4":enum32{"Scan Settings", "MCL FPGA Loop Timing"}(tab)
  out "Total Time (s)":dbl=48.0
  in  "Scan lines (y)":u64=20
  in  "Fast Scan Dir":bool=TRUE
  in  "2D or 1D Scan":bool=TRUE
  out "Initial X":dbl=-1.3598098696859644
  out "Initial Y":dbl=6.297618030335399
  out "Time/f+b scan (s) (MCL)":dbl=2.4 caption="Time/scan (s)"
  in  "Number of scans (MCL)":u64=1 caption="Scans"
  in  "Scan steps (MCL)":u64=40 caption="Scan steps (x)"
  in  "N APD Samp/step":dbl=3.0
  in  "Scan Range (V)\n(of steps)":dbl=3.5
  in  "Restart DMA? (MCL)":bool=TRUE caption="Restart DMA?"
  in  "Continuous MCL Scanning":bool caption="Cont. Scanning"
  in  "Center Scan":bool=TRUE
  in  "Save Data (MCL)":bool=TRUE caption="Save Data"
  out "Actual Incr. int (MCL)":i16=294 caption="Incr. int"
  out "Desired incr (int)":dbl=294.0628205128205
  out "Desired Scan Incr (V)":dbl=0.08974358974358974
  out "N sets should be saved (MCL)":dbl=160.0 caption="N sets should be saved"
  out "Data points/scans (MCL)":dbl=4800.0 caption="Data points/scans"
  out "Data points/scan (f+b)":dbl=240.0 caption="points/scan (f+b)"
  out "Cycles/step (MCL)":u64=2000 caption="Cycles/step" format="%.0p"
  out "Actual MCL Inc (V)":dbl=0.08972441785943175
  in  "Phase adjust (MCL)":i16 caption="Phase adjust"
  out "Relative Phase (MCL)":i16 caption="Relative Phase"
  in  "Initial Phase Adj. (MCL)":i16 caption="Initial Phase Adj."
  in  "Update Count (MCL)":u32=600
  in  "+ phase (MCL)":bool
  in  "- phase (MCL)":bool
  out "MCL Late Counter":u32
  in  "APD 1 AO Mult.":i16=1 min=1
  in  "APD 2 AO Mult.":i16=1 min=1
  in  "Red current when FB OFF (%)":dbl
  in  "Tab Control 7":enum32{"Green FB Signals", "Slow MCL Scan"}(tab)
  out "Green FB Plot":dbl(graph)=-0.008239997558519242
  out "MCL Scan 2":cluster{"Begin (V)":dbl, dbl, dbl[]}(graph)
  out "MCL Scan":cluster{"Begin (V)":dbl, dbl, dbl[]}(graph)
  in  "Green laser mode":enum32{"Laser ON", "Laser OFF", "Interlace"}(radio)=enum."Interlace"
  in  "GI Frequency, ON count":u32=150 min=1 step=1
  in  "Invert GI":bool
  out "GI Late Counter":u32
  in  "Phase adj. (GI)":i16=5
  out "GI relative phase":i16
  in  "+ phase (GI)":bool
  in  "Initial Phase Adjustment (GI)":i16=19
  in  "GI Frequency, OFF count":u32=450 min=1 step=1
  in  "- phase (GI)":bool
  out "Green FB Signals (V)":cluster{"Y":dbl, "X":dbl, "Sum":dbl}={"Y"=-1213.5925925925926, "X"=-1213.5925925925926, "Sum"=-0.008239997558519242}
  out "Relative phase (Green FB)":i16
  in  "+ phase (Green FB)":bool
  in  "- phase (Green FB)":bool
  out "Green FB Count":u32=600
  in  "Phase adj. (Green FB)":i16=10
  in  "Initial Phase Adjustment (Green FB)":i16=50
  in  "Green FB On/Off":bool=TRUE
  in  "Current When FB OFF (%)":dbl=87.0 min=0.0 max=100.0 step=1.0
  in  "Green int current ON count adj":u32=150
  in  "Green FB Gains":T14={"proportional gain (Kc)"=10, "integral gain (Kc*Ts/Ti)"=5, "derivative gain (Kc*Td/Ts)"=0}
  in  "- phase (GI) 2":bool
  in  "Initial Phase Adjustment (GI) 2":i16=-100
  in  "+ phase (GI) 2":bool
  out "GI relative phase 2":i16
  in  "Phase adj. (GI) 2":i16=20
  out "GI Late Counter 2":u32
  in  "On one out of X cycles":u32=1
  in  "Trap Position FIFO Depth":u32=300000 format="%.0p"
  in  "# Samples/trap":u32=20000 format="%.0p"
  out "Trap AI Elements/DMA read":u32=320000 format="%.0p"
  out "Ave. Rate (Hz)":dbl=200000.0 format="%#_6p"
  out "FIFO El. Rem.":u32 format="%.0p"
  in  "Phase adj. (AI1)":i16=15
  out "Relative phase (AI1)":i16
  in  "+ phase (AI1)":bool
  in  "- phase (AI1)":bool
  out "Late Counter (AI1)":u32
  in  "Initial Phase Adjustment (AI1)":i16=220
  out "AI rate (Hz)":dbl=200000.0 format="%#_6p"
  in  "AI Count (ticks)":u32=200
  out "# Samples/channel":u32=40000 format="%.0p"
  in  "Trap AI FIFO Depth":u32=600000 format="%.0p"
  in  "Detector Type":string(combo)="IR-QPD + PSD + FB-QPD X position"
  in  "N Acq Sets (Traps + Fl.)":i16=3
  in  "Sets to FIFO (Traps)":T15={"Set 1"=TRUE, "Set 2"=TRUE, "Set 3"=FALSE}
  in  "FPGA Ave.":dbl=1.0 min=1.0 step=1.0
  out "Ave. Period (s)":dbl=5e-06 format="%#_6p"
  out "DMA Update Period (s)":dbl=0.3
  out "FPGA Averaging":bool
  out "Trap Sets":u32=2
  out "Counts/DMA":dbl=12000000.0 format="%#_6p"
  out "Trap Pos FIFO El Remaining":u32=549
  out "Trap Pos Elements/DMA read":u32=120000 format="%.0p"
  out "Trap AI FIFO Timeout":u16
  out "Trap Pos FIFO Timeout":u16
  in  "Set target":bool
  in  "Target coordinates":cluster{"X1":dbl, "Y1":dbl, "X2":dbl, "Y2":dbl}={"X1"=328.0, "Y1"=274.0, "X2"=368.0, "Y2"=314.0}
  in  "Target size":cluster{"Width":dbl, "Height":dbl}={"Width"=40.0, "Height"=40.0}
  out "Video coordinates":cluster{"X":dbl, "Y":dbl}
  in  "Video Capture Rate (Hz)":dbl=30.0
  in  "Video Index":dbl=1.0 min=1.0 step=1.0
  in  "New Video File":bool
  in  "Save Video":bool
  in  "Reset Averaging":bool
  in  "Averaging":bool
  in  "Save Image":bool
  in  "Image Index":dbl=1.0 min=1.0
  out "Path Out":path
  in  "Center Point":cluster{"X":i32, "Y":i32}={"X"=335, "Y"=271}
  in  "Zoom Factor":sgl=7.0
  out "Window Size":cluster{"Width":i32, "Height":i32}
  out "Window Position":cluster{"X Position":i32, "Y Position":i32}={"X Position"=40, "Y Position"=40}
  in  "Initial Window Size":cluster{"Width":i32, "Height":i32}={"Width"=884, "Height"=619}
  in  "Initial Window Position":cluster{"X Position":i32, "Y Position":i32}={"X Position"=796, "Y Position"=4}
  in  "Intensity Upper":dbl=88.0
  in  "Intensity Lower":dbl=66.0
  out "error out":errorcluster
  out "error out 2":errorcluster
  in  "User":string(combo)
  in  "Load user params":bool
  in  "Save user params":bool
  in  "Bottom  1 Harvard Syringe Pump Serial Port":refnum<visa-resource-name>="COM6"
  in  "Center Harvard Syringe Pump Serial Port":refnum<visa-resource-name>="COM8"
  in  "Lost Tether Alarm Threshold (pN)":dbl=0.5
  in  "AOM X Cal (nm/MHz)":dbl=123.0
  in  "MCL X Cal (nm/V)":dbl=1070.0
  out "X RF Amplitude Limits (%)":T16={"Minimum"=0.0, "Maximum"=50.0, "Increment"=1.0}
  out "X RF Frequency Limits (MHz)":T16={"Minimum"=60.0, "Maximum"=90.0, "Increment"=1.0}
  out "Y RF Frequency Limits (MHz)":T16={"Minimum"=0.0, "Maximum"=40.0, "Increment"=1.0}
  out "Y RF Amplitude Limits (%)":T16={"Minimum"=0.0, "Maximum"=50.0, "Increment"=1.0}
  in  "Manip. X?":bool=TRUE
  in  "Manip. Y?":bool
  in  "Force Manip Abort":bool
  out "Read cal error":errorcluster
  in  "DAQ Delay (ms)":u32=1000
  in  "Start Scan":bool
  in  "Scan axis":bool=TRUE
  in  "Osc. amp. (V)":dbl=5.0
  in  "Osc. center (V)":dbl=5.0
  in  "Osc. freq. (Hz) 2":dbl=1.0
  in  "MCL Mode":u16(ring) items=["Manual Positioning", "Sinusoidal Wave", "Linear Scan"]
  in  "Begin (V)":dbl
  in  "End (V)":dbl=10.0
  in  "N Points":dbl=20.0
  in  "Delay to Interlace (s)":dbl
  in  "Delayed Interlace Start":bool
  in  "Read Lateness and Rel Phase":bool
  out "Vec Mean of T1 T2":dbl[](array[numeric])=[nan, nan]
  in  "Cal read wait (s)":u32=5
  out "Time tether formed":timestamp=timestamp(3419012832.6319866 s since 1904-01-01)
  in  "Sample Chamber Stage Serial Port":refnum<visa-resource-name>="COM3"
  in  "Chemyx Syringe Pump Serial Port":refnum<visa-resource-name>="ASRL3::INSTR"
  in  "Limit Min (MHz)":dbl=10.0 caption="Min (MHz)"
  in  "Limit Max (MHz)":dbl=16.0 caption="Max (MHz)"
  in  "Limits Enable":bool=TRUE caption="Enable"
  out "AI labels":string[](array[string])=["T1 Y", "T1 X", "T1 Sum", "T2 Y", "T2 X", "T2 Sum", "T1 FB X", "T1 FB Sum", "T2 FB X", "T2 FB Sum", "PSD Y", "PSD X", "PSD Y Sum"]
  in  "Save Trap Pos. Data":bool=TRUE
  in  "Lower Ch. Cap.":bool
  in  "Top 3 Harvard Syringe Pump Serial Port":refnum<visa-resource-name>="COM4"
  # "After"
  # "During"
  # "Trap On?"
  # "BD Flow ON?"
  # "Samp Flow ON?"
  # "Fish after\nbreak?"
  # "Thresholds (nm)"
  # "From FX (nm)"
  # "Break?"
  # "Multiple"
  # "Bad fit"
  # "Hysteresis"
  # "Trap Trig. Fl.?"
  # "1"
  # "2"
  # "Fl. Down"
